vi "CC Script Parse Define Exp.vi"(8 "error in (no error)":errorcluster, 9 "To String?":bool, 10 "Exposure in":T1={"Mode"=enum."CDS", "Integration Time"=1.0, "Name"="", "Images"=1} {"Integration Time" format="%.2f"}, 11 "DefineExp Parameters":string="ObjectName \"RA\":\"123.456\",\"DEC\":\"4546.54\"") -> (0 "error out":errorcluster, 1 "Name":string, 2 "Exposure":T1={"Mode"=enum."CDS", "Integration Time"=1.0, "Name"="", "Images"=1} {"Integration Time" format="%#.2f"}, 3 "Script String out":string="ObjectName \"RA\":\"123.456\",\"DEC\":\"4546.54\"")   [LabVIEW 2021]
uses:
  typedefs/CC cluster Exposure.ctl
  Detector/Detector Class/Detector enum Detector Integration Mode.ctl
  <vilib>/regexp/Match Regular Expression.xnode
panel:
  # "DefineExposure \"Name\" Mode=\"xxx\", IntegrationTime=n.nn"
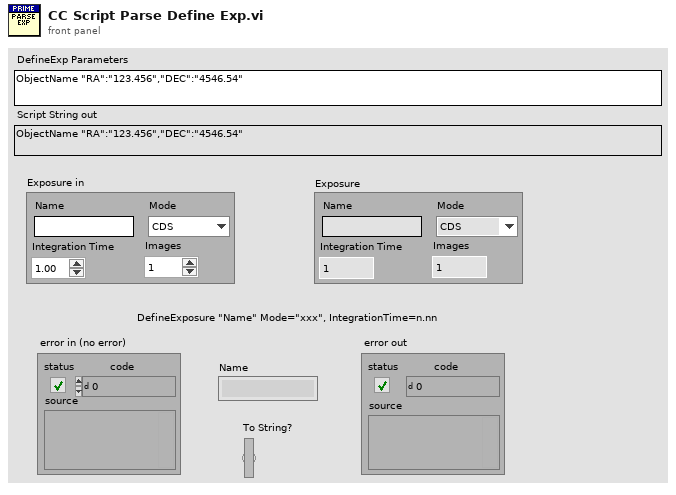
[diagram p1: front panel]
types:
  T1 = typedef "CC cluster Exposure.ctl" = cluster{"Mode":T2, "Integration Time":dbl, "Name":string, "Images":i32}
  T2 = typedef "Detector enum Detector Integration Mode.ctl" = enum16{"SSR", "CDS", "MEAN", "MEDIAN", "MODE", "MIIN", "MAX"}
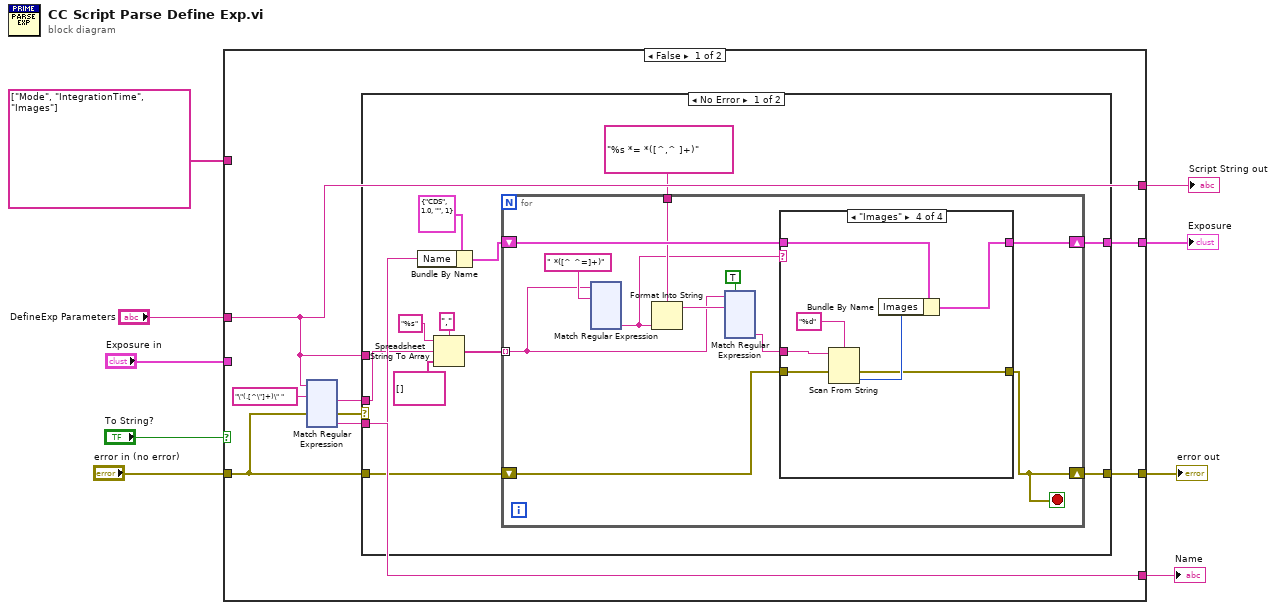
[diagram p0: block diagram]
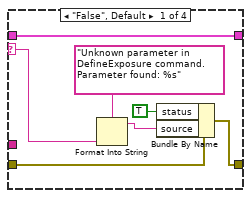
[diagram p2: hidden frame]
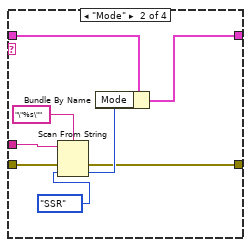
[diagram p3: hidden frame]
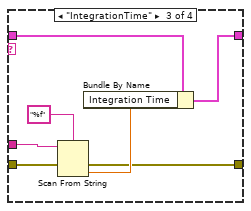
[diagram p4: hidden frame]
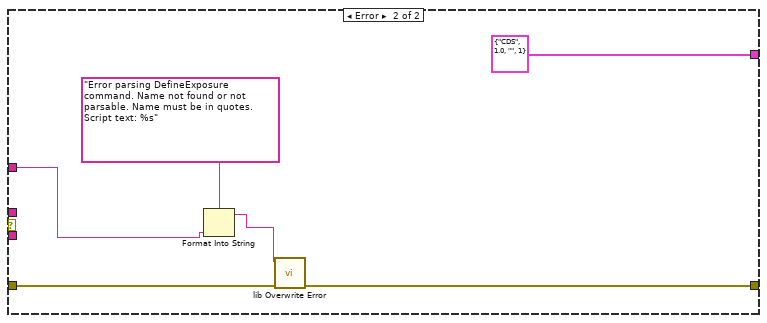
[diagram p5: hidden frame]
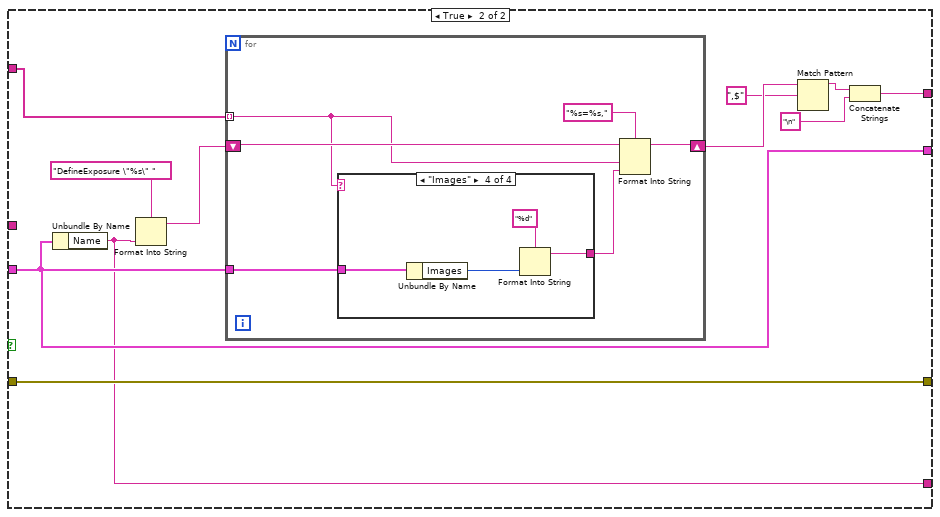
[diagram p6: hidden frame]
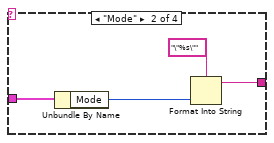
[diagram p8: hidden frame]
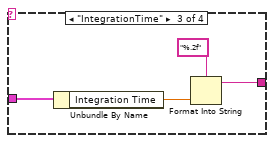
[diagram p9: hidden frame]
diagram:
  n1 = case shown="False" "To String?" {
    tunnel: "DefineExp Parameters" -> [w10 _]
    tunnel: string[] ["Mode", "IntegrationTime", "Images"] -> [_ w437]
    tunnel: [w16 w434] -> w7
    tunnel: "error in (no error)" -> [w12 w436]
    tunnel: [w15 w436] -> w5
    tunnel: "Exposure in" -> [_ w434]
    tunnel: [w10 w435] -> w2
    tunnel: [w14 w433] -> w1
    frame False {
      n2 = xnode "Match Regular Expression"("input string"=w10, "regular expression"="\"(.[^\"]+)\" ", "error in"=w12) -> ("after match"=w13:string, "error out"=w11:errorcluster, "submatch 1"=w14:string)  [unwired: 3 in, 3 out]
      n3 = case shown="No Error" w11 {
        tunnel: [w27 T1 {"Mode"=enum."CDS", "Integration Time"=1.0, "Name"="", "Images"=1} ("Exposure")] -> w16
        tunnel: [w26 w309] -> w15
        tunnel: w14 -> [w25 _]
        tunnel: w13 -> [w21 _]
        tunnel: w12 -> [w18 w310]
        tunnel: w10 -> [_ w312]
        frame No Error {
          n4 = Bundle By Name(cluster=T1 {"Mode"=enum."CDS", "Integration Time"=1.0, "Name"="", "Images"=1} ("Exposure"), "Name"=w25) -> (w29:T1)
          n5 = Spreadsheet String To Array(delimiter (Tab)=",", format string="%s", spreadsheet string=w21, array type (2D Dbl)=string[] []) -> (array=w20:string[])
          n6 = for {
            tunnel: w20 -> [w33] mode=indexing
            shift-right: [w39] -> w27
            shift-left: w29 -> [w40]
            shift-right: [w30] -> w26
            shift-left: w18 -> [w38]
            tunnel: "%s *= *([^,^ ]+)" ("regular expression") -> [w35]
            stop <- w30 stop-if-true
            n7 = xnode "Match Regular Expression"("input string"=w33, "regular expression"=" *([^ ^=]+)" ("format string")) -> ("submatch 1"=w32:string)  [unwired: 4 in, 5 out]
            n8 = Format Into String(format string=w35, w32) -> (resulting string=w37:string)  [unwired: 2 in, 1 out]
            n9 = xnode "Match Regular Expression"("input string"=w33, "regular expression"=w37, "ignore case? (F)"=TRUE) -> ("submatch 1"=w31:string)  [unwired: 3 in, 5 out]
            n10 = case shown="\"Images\"" w32 {
              selector: w32 -> [w283 _ _ _]
              tunnel: w40 -> [w285 w293 w300 w307]
              tunnel: w31 -> [_ w291 w298 w305]
              tunnel: [w285 w289 w297 w304] -> w39
              tunnel: w38 -> [w282 w288 w295 w302]
              tunnel: [w279 w287 w294 w301] -> w30
              frame "False", Default {
                n11 = Format Into String(format string="Unknown parameter in DefineExposure command. Parameter found: %s", w283) -> (resulting string=w281:string)  [unwired: 2 in, 1 out]
                n12 = Bundle By Name(cluster=w282, "status"=TRUE, "source"=w281) -> (w279:errorcluster)
              }
              frame "Mode" {
                n13 = Scan From String(format string="\"%s\"", input string=w291, error in=w288, default 1=Detector_enum_Detector_Integration_Mode."SSR" ("Mode")) -> (error out=w287:errorcluster, output 1=w290:T2)  [unwired: 1 in, 2 out]
                n14 = Bundle By Name(cluster=w293, "Mode"=w290) -> (w289:T1)
              }
              frame "IntegrationTime" {
                n15 = Scan From String(format string="%f", input string=w298, error in=w295) -> (error out=w294:errorcluster, output 1=w296:dbl)  [unwired: 2 in, 2 out]
                n16 = Bundle By Name(cluster=w300, "Integration Time"=w296) -> (w297:T1)
              }
              frame "Images" {
                n17 = Scan From String(format string="%d", input string=w305, error in=w302) -> (error out=w301:errorcluster, output 1=w303:i32)  [unwired: 2 in, 2 out]
                n18 = Bundle By Name(cluster=w307, "Images"=w303) -> (w304:T1)
              }
            }
          }
        }
        frame Error {
          n19 = Format Into String(format string="Error parsing DefineExposure command. Name not found or not parsable. Name must be in quotes. Script text: %s", w312) -> (resulting string=w311:string)  [unwired: 2 in, 1 out]
          n20 = call "lib Overwrite Error.vi"("error in (no error)"=w310, "Error Message"=w311) -> ("error out"=w309:errorcluster)  [unwired: 9 in]
        }
      }
    }
    frame True {
      n21 = Unbundle By Name(w434) -> ("Name"=w433:string)
      n22 = Format Into String(format string="DefineExposure \"%s\" ", w433) -> (resulting string=w442:string)  [unwired: 2 in, 1 out]
      n23 = for {
        tunnel: w437 -> [w446] mode=indexing
        shift-right: [w444] -> w441
        shift-left: w442 -> [w448]
        tunnel: w434 -> [w449]
        n24 = case shown="\"Images\"" w446 {
          tunnel: w449 -> [_ w453 w457 w461]
          tunnel: [_ w450 w454 w458] -> w445
          frame "False", Default {
          }
          frame "Mode" {
            n25 = Unbundle By Name(w453) -> ("Mode"=w451:T2)
            n26 = Format Into String(format string="\"%s\"", w451) -> (resulting string=w450:string)  [unwired: 2 in, 1 out]
          }
          frame "IntegrationTime" {
            n27 = Unbundle By Name(w457) -> ("Integration Time"=w455:dbl)
            n28 = Format Into String(format string="%.2f", w455) -> (resulting string=w454:string)  [unwired: 2 in, 1 out]
          }
          frame "Images" {
            n29 = Unbundle By Name(w461) -> ("Images"=w459:i32)
            n30 = Format Into String(format string="%d", w459) -> (resulting string=w458:string)  [unwired: 2 in, 1 out]
          }
        }
        n31 = Format Into String(format string="%s=%s,", initial string=w448, w446, w445) -> (resulting string=w444:string)  [unwired: 1 in, 1 out]
      }
      n32 = Match Pattern(string=w441, regular expression=",$") -> (before substring=w439:string)  [unwired: 1 in, 3 out]
      n33 = Concatenate Strings(w439, "\n" ("string")) -> (w435:string)
    }
  }
  "error out" <- w5
  "Exposure" <- w7
  "Script String out" <- w2
  "Name" <- w1
